vi "DMM_Scan PRD 32V-16C Initialize.vi"(0 "Scan Resource Names":T6={"DMM Resource Name"="DMM_4065", "MUX and Shunt Resource Name"="MUX_2567"}, 2 "Powerline Frequency":T7=enum."50 Hz", 5 "Topology":T2={"MUX Topology Name"="2567/Independent"}, 7 "Close all Shunts?":bool=TRUE, 9 "Relay Debounce Time (ms)":u32=5, 11 "error in":errorcluster) -> (4 "Scan Resource Handles out":T1={"DMM Handle"="", "MUX Handle"="", "Relays Debounce Time (ms)"=5, "Close all Shunts?"=TRUE}, 6 "Switches Characteristics":T4, 15 "error out":errorcluster)   [LabVIEW 2021, in "DMM_Scan PXI RLY Driver 32V-16C.lvlib"]
doc: "Creates a new NI-DMM Scan driver session on each device specified in the Scan Resource Names control configured with the local powerline frequency. The devices use the powerline frequency value to select a timebase for setting the Aperture Time property in powerline cycles (PLCs). Change Powerline Frequency value to 60 Hz for North & South America.\n\nA specific switch topology associated to a fixed hardware mapping channels defined by default for the random maximum 32 voltages and 16 currents configuration. Each channel number for current is linked to the same channel shunt number +16 starting from ch32. (ex. Current ch32 linked to Shunt ch48, ch33 linked to ch49...)\n\n- \"Close all Shunts\" input is used to close all shunts relays from channels 48 to 63 (NI 2567) from the fixed Channels Topology Mapping, allowing to continuously powerthe DUT during all measurements.\n\nDeselect \"Close all shunts\" optionally to open current shunts. For example, in the event a 2-Wire Resistance measurement function without any current through the DUT is desired.\n\n- Relays Debounce Time (ms), defines the timing specifications for the external relays debounce time. Typical default Value is 5 ms, but needs to be adjusted with you specific choice of external relays. \n\nThe VI returns the switch max voltage and current characteristics from multiplexer and shunt relays, but only if the NI Multiplexer use embedded relays. The values will be 0 for external custom relays as for the NI 2567 Relay Driver only."
uses:
  DMM_Scan PXI RLY Driver 32V-16C.lvlib
  <instrlib>/niDMM/nidmm.llb/niDMM Powerline Frequency.ctl
  Typedefs/Scan Resource Names.ctl
  Typedefs/Switches Characteristics.ctl
  Static Digital Path Generation/Typedefs/Module Characteristics.ctl
  Typedefs/Topology.ctl
  <instrlib>/niSwitch/niSwitch.llb/niSwitch Topologies.ctl
  Typedefs/Scan Resource Handles Out.ctl
  Static Digital Path Generation/Typedefs/Terminal and State Settings.ctl
  DMM Mixed Measurements/DMM_Mixed Measurement.lvlib
  Static Digital Path Generation/Switch_Static Digital Path Generation.lvlib
panel:
  # "Inputs"
  # "Outputs"
  # "Overview:\nThis VI interacts with the NI-DMM and NI-SWITCH drivers to initialize NI-DMM instruments and provide a corresponding instrument handle according to the topology selected. It also utilized a fixed hardware mapping topology from the Independent Relay Multiplexer (ex. NI PXI-2567) you will use.\n\nHardware Requirements: A PXI, PCIe, or USB DMM instrument, any Switch with the same topology as NI PXI-2567 Independent Relay. Need external relays DPST for 2-wire (Differential) measurements.\n\nSoftware Requirements: NI-DMM 2022 Q3 or above, NI-SWITCH 2022 Q4 or above\n\nInstructions:\nSelect your DMM instrument resource name in the drop down control\nSelect your Multiplexer Switch resource (Will be partially used for the Shunt Relays)\nSelect the topology for channel mapping. Default is \"2567/Independent\"\nSelect your Power Line Frequency (Default 50 Hz) and deselect the \"Close all Shunts?\"boolean (Default ON) if you don't need to power your DUT through Current Shunt relays.\n\nNote: each \"DMM Handle Out\" indicator will be used by the Configure & Measure and Close API functions"
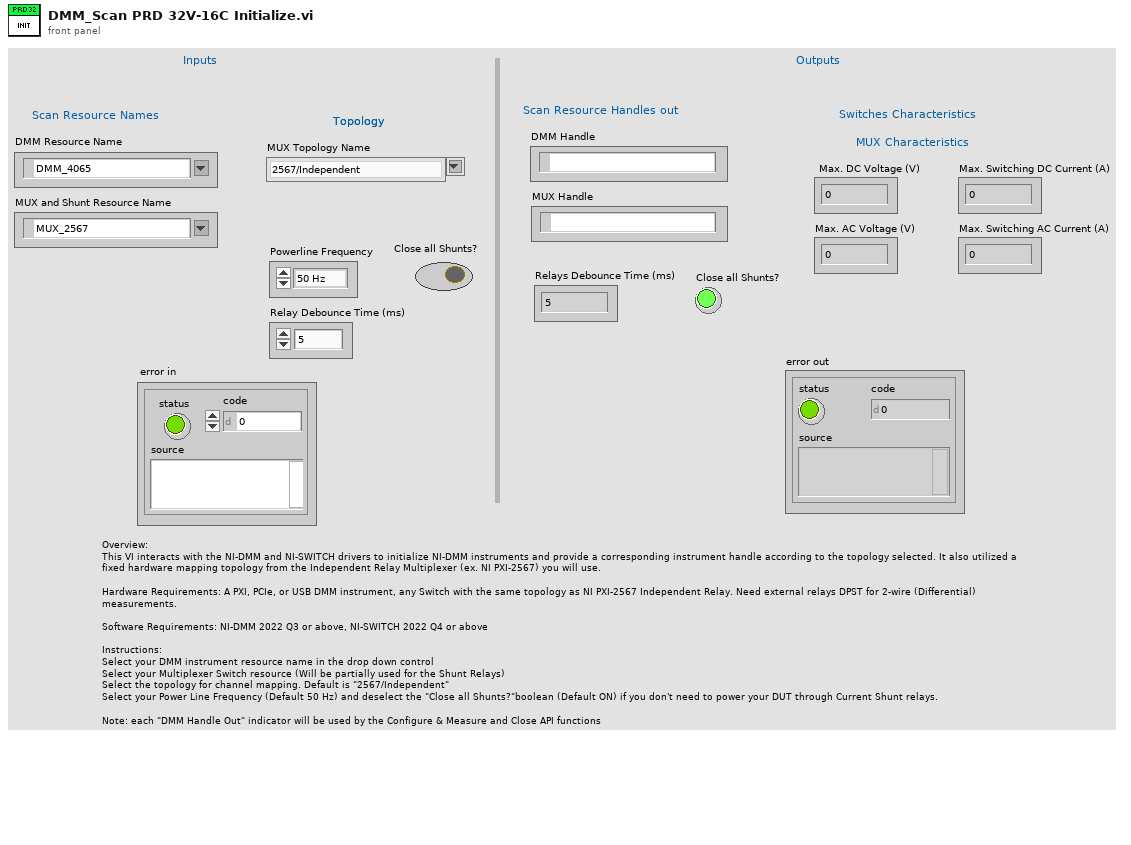
[diagram p1: front panel]
types:
  T1 = typedef "DMM_Scan PXI RLY Driver 32V-16C.lvlib/Scan Resource Handles Out.ctl" = cluster{"DMM Handle":refnum<k15>, "MUX Handle":refnum<k15>, "Relays Debounce Time (ms)":u32, "Close all Shunts?":bool}
  T2 = typedef "DMM_Scan PXI RLY Driver 32V-16C.lvlib/Topology.ctl" = cluster{"MUX Topology Name":T3}
  T3 = typedef "niSwitch Topologies.ctl" = string
  T4 = typedef "DMM_Scan PXI RLY Driver 32V-16C.lvlib/Switches Characteristics.ctl" = cluster{"Mux Characteristics":T5}
  T5 = typedef "Switch_Static Digital Path Generation.lvlib/Module Characteristics.ctl" = cluster{" Max. DC Voltage (V)":dbl, "Max. Switching DC Current (A)":dbl, "Max. AC Voltage (V)":dbl, "Max. Switching AC Current (A)":dbl}
  T6 = typedef "DMM_Scan PXI RLY Driver 32V-16C.lvlib/Scan Resource Names.ctl" = cluster{"DMM Resource Name":refnum<k15>, "MUX and Shunt Resource Name":refnum<k15>}
  T7 = typedef "niDMM Powerline Frequency.ctl" = enum16{"60 Hz", "50 Hz"}
  T8 = typedef "Switch_Static Digital Path Generation.lvlib/Terminal and State Settings.ctl" = cluster{"Connect/Disconnect":bool, "Channel 1":string, "Channel 2":string}
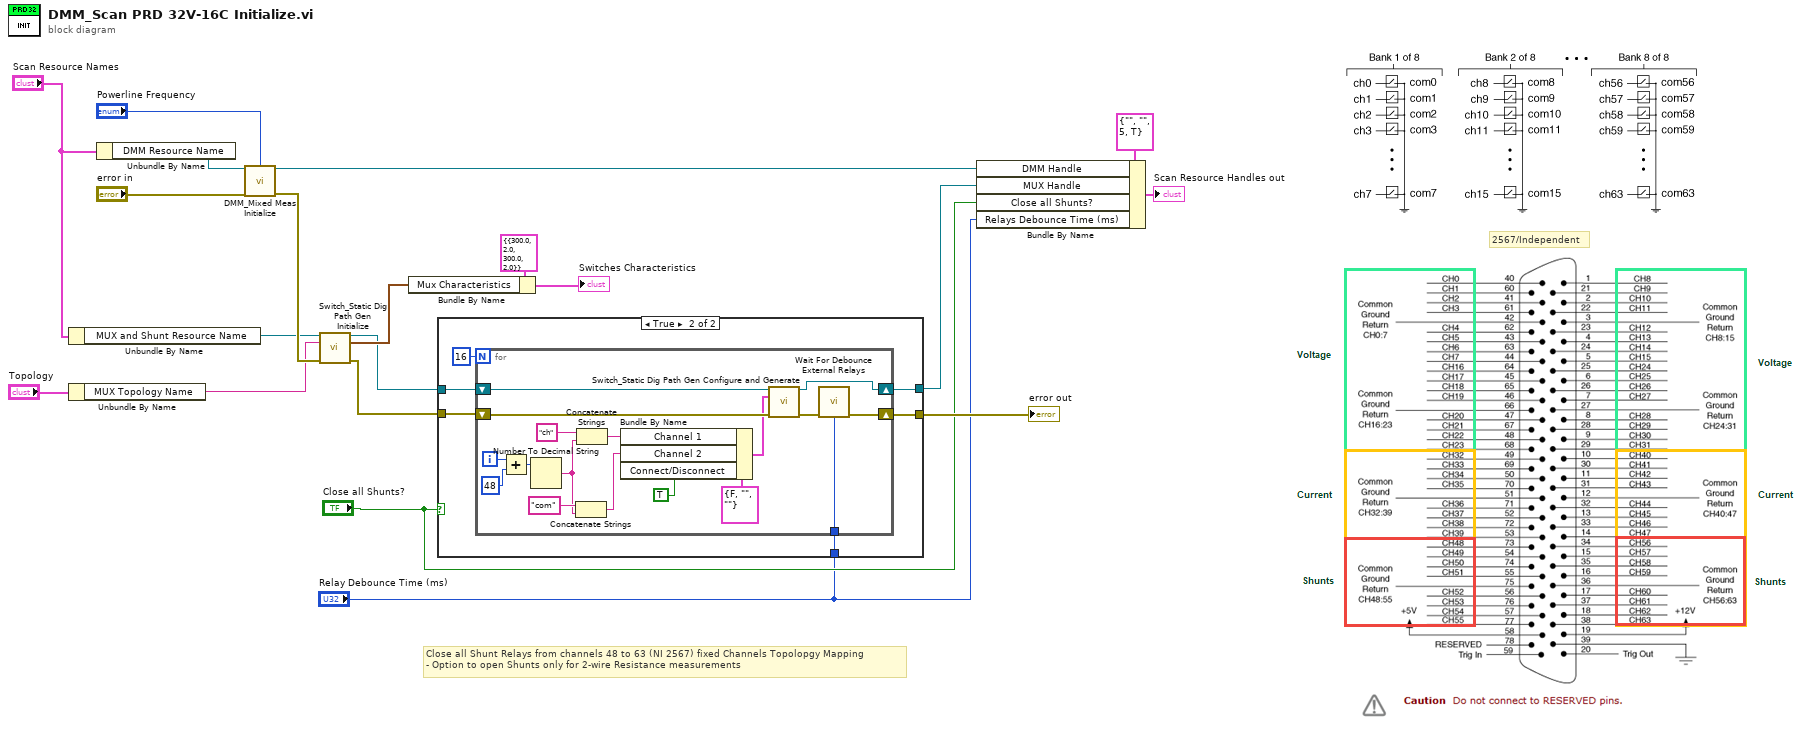
[diagram p0: block diagram]
diagram:
  # "Close all Shunt Relays from channels 48 to 63 (NI 2567) fixed Channels Topolopgy Mapping\n- Option to open Shunts only for 2-wire Resistance measurements"
  # "2567/Independent"
  n1 = Unbundle By Name("Scan Resource Names") -> ("MUX and Shunt Resource Name"=w14:refnum<k15>)
  n2 = Unbundle By Name("Topology") -> ("MUX Topology Name"=w17:T3)
  n3 = Unbundle By Name("Scan Resource Names") -> ("DMM Resource Name"=w15:refnum<k15>)
  n4 = call "DMM_Mixed Meas Initialize.vi"("DMM Resource Name"=w15, "Powerline Frequency"="Powerline Frequency", "error in"="error in") -> ("DMM Handle Out"=w13:refnum<k15>, "error out"=w20:errorcluster)  [unwired: 11 in]
  n5 = call "Switch_Static Dig Path Gen Initialize.vi"("Switch Resource Name"=w14, "Topology Name"=w17, "error in"=w20) -> ("Switch Handle Out"=w8:refnum<k15>, "Module Characteristics"=w16:T5, "error out"=w7:errorcluster)  [unwired: 10 in]
  n6 = Bundle By Name(cluster=T4 {"Mux Characteristics"={" Max. DC Voltage (V)"=300.0, "Max. Switching DC Current (A)"=2.0, "Max. AC Voltage (V)"=300.0, "Max. Switching AC Current (A)"=2.0}} ("Switches Characteristics"), "Mux Characteristics"=w16) -> (→"Switches Characteristics":T4)
  n7 = case shown="True" "Close all Shunts?" {
    tunnel: w8 -> [w22 w28]
    tunnel: [w22 w27] -> w6
    tunnel: w7 -> [w21 w26]
    tunnel: [w21 w25] -> w5
    tunnel: "Relay Debounce Time (ms)" -> [_ w23]
    frame False {
    }
    frame True {
      n8 = for {
        N: 16 -> [_]
        shift-right: [w31] -> w27
        shift-left: w28 -> [w45]
        shift-right: [w30] -> w25
        shift-left: w26 -> [w44]
        tunnel: w23 -> [w29]
        i -> [w43]
        n9 = Add(x=w43, y=48) -> (x+y=w41:i32)
        n10 = Number To Decimal String(number=w41) -> (decimal integer string=w34:string)  [unwired: 1 in]
        n11 = Concatenate Strings("com" ("string"), w34) -> (w33:string)
        n12 = Concatenate Strings("ch" ("string"), w34) -> (w36:string)
        n13 = Bundle By Name(cluster=T8 {"Connect/Disconnect"=FALSE, "Channel 1"="", "Channel 2"=""} ("Terminal and State Settings"), "Channel 1"=w36, "Channel 2"=w33, "Connect/Disconnect"=TRUE) -> (w40:T8)
        n14 = call "Switch_Static Dig Path Gen Configure and Generate.vi"("Switch Handle In"=w45, "Terminal and State Settings"=w40, "error in"=w44) -> ("Switch Handle Out"=w31:refnum<k15>, "error out"=w32:errorcluster)  [unwired: 10 in, 1 out]
        n15 = call "Wait For Debounce External Relays.vi"("error in"=w32, "Wait (ms)"=w29) -> ("error out"=w30:errorcluster)  [unwired: 13 in]
      }
    }
  }
  "error out" <- w5
  n16 = Bundle By Name(cluster=T1 {"DMM Handle"="", "MUX Handle"="", "Relays Debounce Time (ms)"=5, "Close all Shunts?"=TRUE} ("Scan Resources Handles Out"), "DMM Handle"=w13, "MUX Handle"=w6, "Close all Shunts?"="Close all Shunts?", "Relays Debounce Time (ms)"="Relay Debounce Time (ms)") -> (→"Scan Resource Handles out":T1)
